vi "Sets_Diff(CDB).vi"(8 "error in (no error)":errorcluster caption="错误输入（无错误）", 10 "输入数组B":cdb[](array[numeric]), 11 "输入数组A":cdb[](array[numeric])) -> (0 "error out":errorcluster caption="错误输出", 2 "数组C索引":i32[](array[numeric]), 3 "输出数组C":cdb[](array[numeric]) format="%.2f")   [LabVIEW 2012]
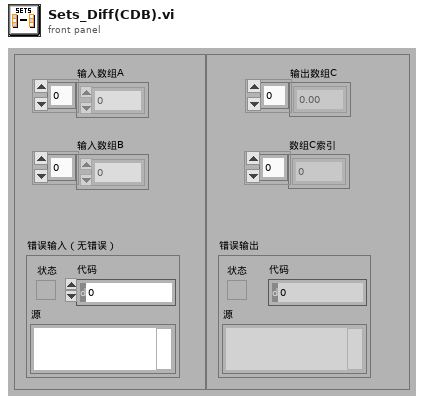
[diagram p1: front panel]
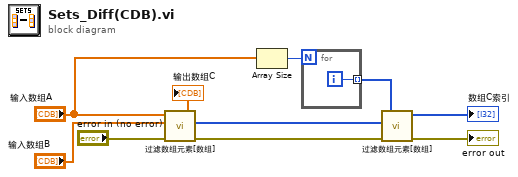
[diagram p0: block diagram]
diagram:
  n1 = call-poly "过滤数组元素[数组].vi"("error in (no error)"="error in (no error)", "过滤元素"="输入数组B", "输入数组"="输入数组A") -> ("error out"=w6:errorcluster, "已过滤元素索引"=w2:i32[], "输出数组"=→"输出数组C":cdb[])  [unwired: 6 in]
  n2 = Array Size(array="输入数组A") -> (size(s)=w10:i32)
  n3 = for {
    N: w10 -> [_]
    tunnel: [w11] -> w9 mode=indexing
    i -> [w11]
  }
  n4 = call-poly "过滤数组元素[数组].vi"("error in (no error)"=w6, "过滤元素"=w2, "输入数组"=w9) -> ("error out"=→"error out":errorcluster, "输出数组"=→"数组C索引":i32[])  [unwired: 6 in, 1 out]
